vi "Add Record.vi"(8 "error in":errorcluster, 10 "Records":refnum<class "Record.lvclass">, 11 "Structure in":refnum<class "Structure.lvclass">) -> (0 "error out":errorcluster, 3 "Structure out":refnum<class "Structure.lvclass">)   [LabVIEW 2019, in "Structure.lvclass"]
uses:
  Structure.lvclass
  Record/Record.lvclass
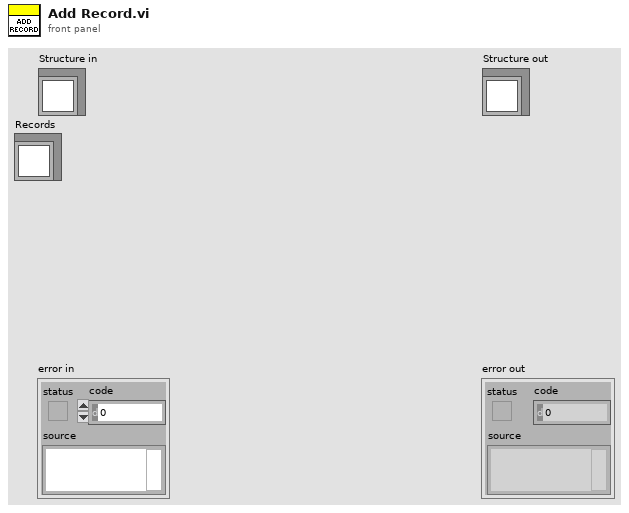
[diagram p1: front panel]
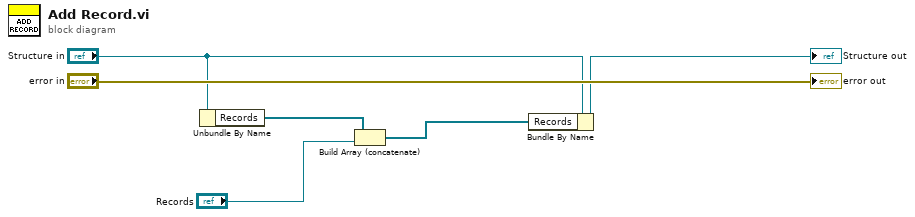
[diagram p0: block diagram]
diagram:
  n1 = Unbundle By Name("Structure in") -> ("Records"=w2:refnum<class "Record.lvclass">[])
  n2 = Build Array (concatenate)(w2, "Records") -> (w1:refnum<class "Record.lvclass">[])
  n3 = Bundle By Name(cluster="Structure in", "Records"=w1) -> (→"Structure out":refnum<class "Structure.lvclass">)
  "error out" <- "error in"
